vi "Enk Data przenies FVG.vi"(7 "Akcja (SET)":T2=enum."SET", 8 "error in (no error)":errorcluster, 11 "Enkoder Data in":T1) -> (0 "error out":errorcluster, 3 "Enkoder Data out":T1)   [LabVIEW 2014]
doc: "Use this template to build a VI to use as a subVI."
uses:
  Kontrolki/GUI/Enkoder Data.ctl
  Kontrolki/FVGs/FVG akcje podstawowa.ctl
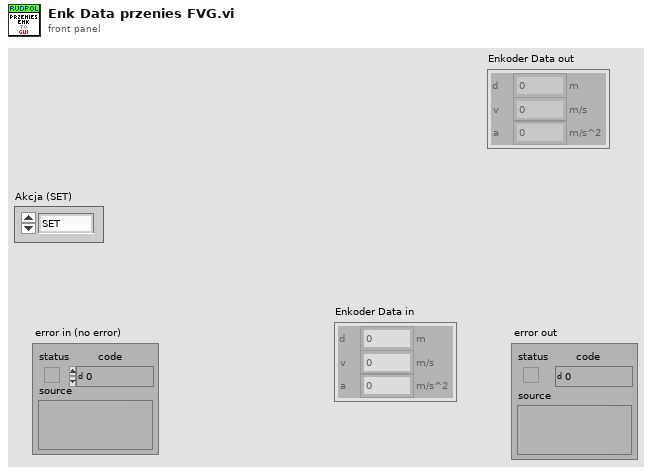
[diagram p1: front panel]
types:
  T1 = typedef "Enkoder Data.ctl" = cluster{"d":dbl, "v":dbl, "a":dbl}
  T2 = typedef "FVG akcje podstawowa.ctl" = enum16{"GET", "SET"}
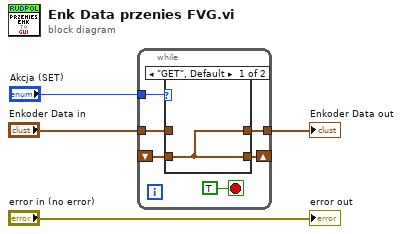
[diagram p0: block diagram]
diagram:
  n1 = while {
    shift-right: [w7] -> _
    shift-left: _ -> [w6]
    tunnel: "Akcja (SET)" -> [w9]
    tunnel: [w8] -> w2
    tunnel: "Enkoder Data in" -> [w5]
    stop <- TRUE stop-if-true
    n2 = case shown="\"GET\", Default" w9 {
      tunnel: [w11 w12] -> w8
      tunnel: [w11 w12] -> w7
      tunnel: w6 -> [w11 _]
      tunnel: w5 -> [_ w12]
      frame "GET", Default {
      }
      frame "SET" {
      }
    }
  }
  "Enkoder Data out" <- w2
  "error out" <- "error in (no error)"
